vi "Untitled 1222222.vi"() -> ()   [LabVIEW 2010]
uses:
  <vilib>/NXT/Block Support/NXT_InputPort.ctl
  <vilib>/NXT/Subs/MotorOutput.ctl
  <vilib>/NXT/Dual Mode Library/Sensors/Light_Off.vi
  <vilib>/NXT/Dual Mode Library/Motors/MotorOn.vi
  <vilib>/NXT/Dual Mode Library/Motors/MotorBrake.vi
panel:
  in  "stop":bool
  in  "c":T1=3 items=["Port A", "Port B", "Port C", "All Ports"]
  in  "a":T1=3 items=["Port A", "Port B", "Port C", "All Ports"]
  in  "Output Port (All Ports)":T1=3 items=["Port A", "Port B", "Port C", "All Ports"]
  in  "Power (75)":i32=75
  in  "4锅":T2 items=["Port 1", "Port 2", "Port 3", "Port 4"]
  in  "1":T2 items=["Port 1", "Port 2", "Port 3", "Port 4"]
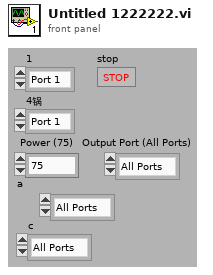
[diagram p1: front panel]
types:
  T1 = typedef "MotorOutput.ctl" = u8
  T2 = typedef "NXT_InputPort.ctl" = u8
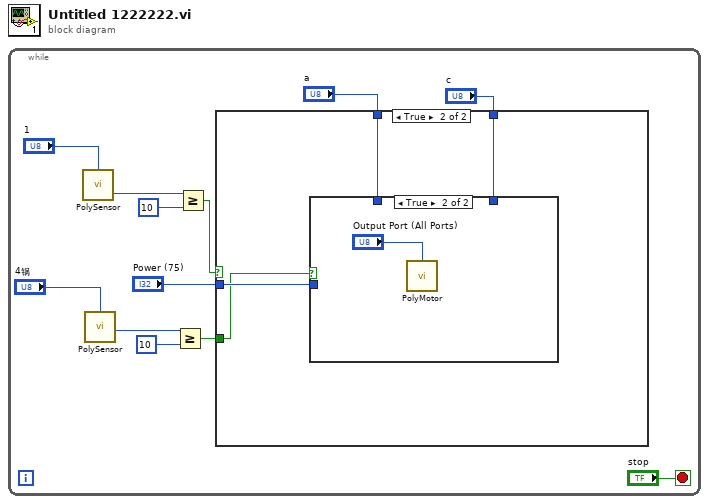
[diagram p0: block diagram]
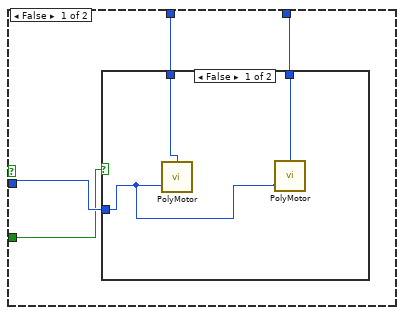
[diagram p2: hidden frame]
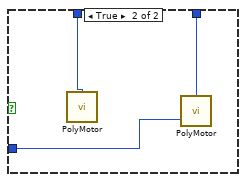
[diagram p3: hidden frame]
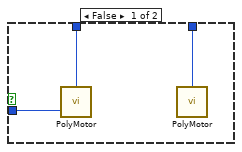
[diagram p4: hidden frame]
diagram:
  n1 = while {
    stop <- "stop" stop-if-true
    n2 = call-poly <vilib>:"PolySensor.vi"("Port (Port 3)"="1") -> ("Scaled Value"=w6:i16)  [unwired: 2 in, 1 out]
    n3 = call-poly <vilib>:"PolySensor.vi"("Port (Port 3)"="4锅") -> ("Scaled Value"=w8:i16)  [unwired: 2 in, 1 out]
    n4 = Greater Or Equal?(x=w8, y=i16 10 ("Scaled Value")) -> (x >= y?=w2:bool)
    n5 = Greater Or Equal?(x=w6, y=i16 10 ("Scaled Value")) -> (x >= y?=w1:bool)
    n6 = case shown="True" w1 {
      tunnel: "Power (75)" -> [w14 w26]
      tunnel: "a" -> [w16 w25]
      tunnel: "c" -> [w15 w24]
      tunnel: w2 -> [w13 w23]
      frame False {
        n7 = case shown="False" w13 {
          tunnel: w16 -> [w19 w22]
          tunnel: w15 -> [w18 w21]
          tunnel: w14 -> [w17 w20]
          frame False {
            n8 = call-poly <vilib>:"PolyMotor.vi"("Power (75)"=w17, "Output Port (All Ports)"=w19) -> ()  [unwired: 2 in, 1 out]
            n9 = call-poly <vilib>:"PolyMotor.vi"("Power (75)"=w17, "Output Port (All Ports)"=w18) -> ()  [unwired: 2 in, 1 out]
          }
          frame True {
            n10 = call-poly <vilib>:"PolyMotor.vi"("Port (All Ports)"=w22) -> ()  [unwired: 3 in, 1 out]
            n11 = call-poly <vilib>:"PolyMotor.vi"("Power (75)"=w20, "Output Port (All Ports)"=w21) -> ()  [unwired: 2 in, 1 out]
          }
        }
      }
      frame True {
        n12 = case shown="True" w23 {
          tunnel: w26 -> [w27 _]
          tunnel: w25 -> [w29 _]
          tunnel: w24 -> [w28 _]
          frame False {
            n13 = call-poly <vilib>:"PolyMotor.vi"("Power (75)"=w27, "Output Port (All Ports)"=w29) -> ()  [unwired: 2 in, 1 out]
            n14 = call-poly <vilib>:"PolyMotor.vi"("Port (All Ports)"=w28) -> ()  [unwired: 3 in, 1 out]
          }
          frame True {
            n15 = call-poly <vilib>:"PolyMotor.vi"("Port (All Ports)"="Output Port (All Ports)") -> ()  [unwired: 3 in, 1 out]
          }
        }
      }
    }
  }
